vi "Configure Roscillator.vi"(7 "Enable Auto Source (T: Enable)":bool=TRUE, 8 "error in (no error)":errorcluster, 9 "Oscillator Source (0: Internal )":i32(ring) items=["Internal ", "External"], 10 "External Frequency (1E7 Hz)":dbl(ring)=10000000.0 items=["1E6"=1000000.0, "5E6"=5000000.0, "1E7"=10000000.0], 11 "VISA resource name":refnum<visa-resource-name>) -> (0 "error out":errorcluster, 3 "VISA resource name out":refnum<visa-resource-name>)   [LabVIEW 2021, in "Agilent 532XX Series.lvlib"]
doc: "Configures the characteristics of the roscillator system."
uses:
  <instrlib>/Agilent 532XX Series/Agilent 532XX Series.lvlib
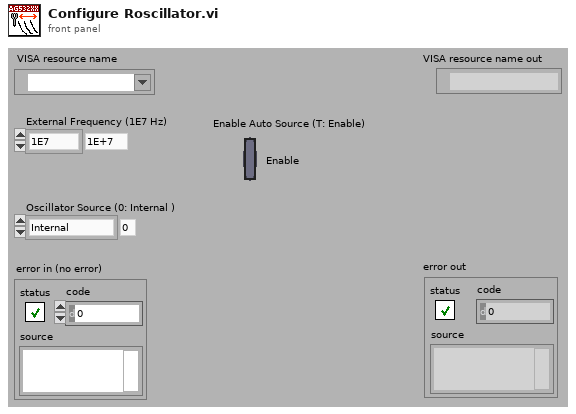
[diagram p1: front panel]
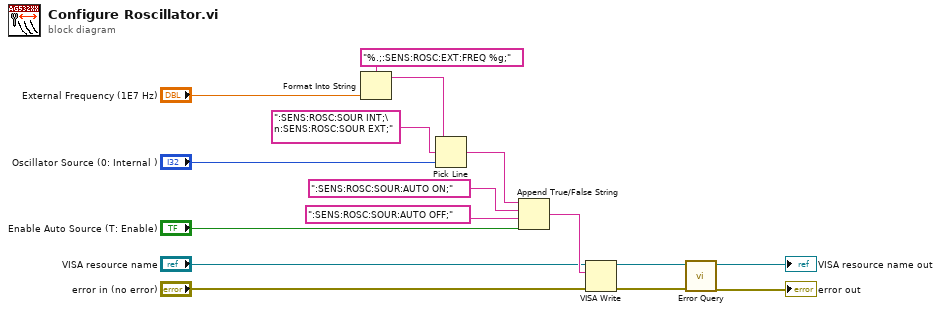
[diagram p0: block diagram]
diagram:
  n1 = Format Into String(format string="%.;:SENS:ROSC:EXT:FREQ %g;", "External Frequency (1E7 Hz)") -> (resulting string=w12:string)  [unwired: 2 in, 1 out]
  n2 = Pick Line(string ("")=w12, multi-line string=":SENS:ROSC:SOUR INT;\n:SENS:ROSC:SOUR EXT;", line index="Oscillator Source (0: Internal )") -> (output string=w11:string)
  n3 = Append True/False String(1:"Enable Auto Source (T: Enable)", 2:":SENS:ROSC:SOUR:AUTO OFF;", 3:":SENS:ROSC:SOUR:AUTO ON;", 4:w11) -> (0:w8:string)
  n4 = VISA Write(VISA resource name="VISA resource name", write buffer=w8, error in (no error)="error in (no error)") -> (VISA resource name out=w5:refnum<visa-resource-name>, error out=w4:errorcluster)  [unwired: 1 out]
  n5 = call <instrlib>:"Error Query.vi"("error in (no error)"=w4, "VISA resource name"=w5) -> ("error out"=→"error out":errorcluster, "VISA resource name out"=→"VISA resource name out":refnum<visa-resource-name>)  [unwired: 8 out]
